vi "Create UI Events.vi"(8 "error in (no error)":errorcluster) -> (0 "error out":errorcluster, 2 "UI Events":T1)   [LabVIEW 2015, in "Simple Progress Bar.lvlib"]
uses:
  Simple Progress Bar.lvlib
  UI Events.ctl
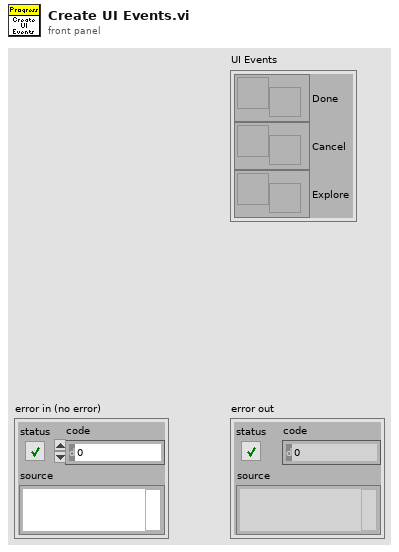
[diagram p1: front panel]
types:
  T1 = typedef "Simple Progress Bar.lvlib/UI Events.ctl" = cluster{"Done":refnum<user-event>, "Cancel":refnum<user-event>, "Explore":refnum<user-event>}
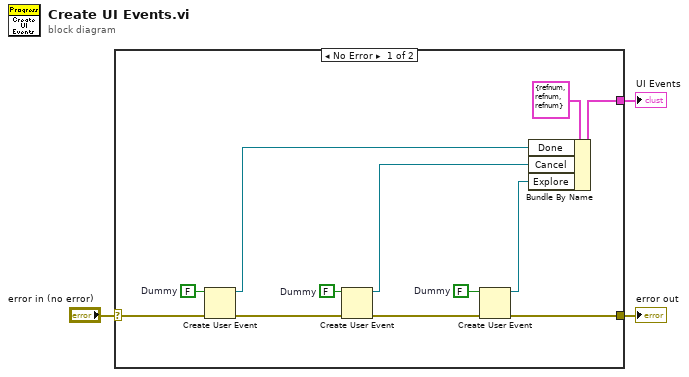
[diagram p0: block diagram]
diagram:
  n1 = case shown="No Error" "error in (no error)" {
    selector: "error in (no error)" -> [w12 w16]
    tunnel: [w4 w16] -> w2
    tunnel: [w13 _] -> w1
    frame No Error {
      w10 = FALSE  # Dummy
      w9 = FALSE  # Dummy
      w15 = FALSE  # Dummy
      n2 = Create User Event(user event datatype=w15, error in=w12) -> (user event=w11:refnum<user-event>, error out=w8:errorcluster)
      n3 = Create User Event(user event datatype=w9, error in=w8) -> (user event=w6:refnum<user-event>, error out=w7:errorcluster)
      n4 = Create User Event(user event datatype=w10, error in=w7) -> (user event=w5:refnum<user-event>, error out=w4:errorcluster)
      n5 = Bundle By Name(cluster=T1 {"Done"=refnum, "Cancel"=refnum, "Explore"=refnum} ("UI Events"), "Done"=w11, "Cancel"=w6, "Explore"=w5) -> (w13:T1)
    }
    frame Error {
    }
  }
  "error out" <- w2
  "UI Events" <- w1
